vi "Calculate Percentage of each Element in Array.vi"(1 "[Count]":i32[](array[numeric])) -> (0 "[% Count\\":dbl[](array[numeric]))   [LabVIEW 2012]
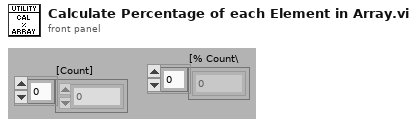
[diagram p1: front panel]
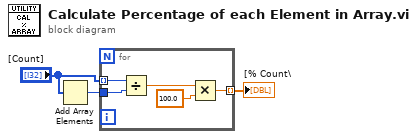
[diagram p0: block diagram]
diagram:
  n1 = Add Array Elements(numeric array="[Count]") -> (sum=w2:i32)
  n2 = for {
    tunnel: "[Count]" -> [w8] mode=indexing
    tunnel: [w5] -> w1 mode=indexing
    tunnel: w2 -> [w4]
    n3 = Divide(x=w8, y=w4) -> (x/y=w7:dbl)
    n4 = Multiply(x=w7, y=100.0) -> (x*y=w5:dbl)
  }
  "[% Count\\" <- w1
